vi "Litho Interpolater_shicheng.vi"(3 "Function generator":T1(array[cluster]) {"square wave duty cycle (%)" format="%0.2f"}, 4 "Lithography Data In":T2(array[cluster]), 5 "Distance":dbl) -> (0 "XY Graph":cluster{dbl[], "Y":dbl[]}(graph), 1 "Simulator Data Out":T3(array[cluster]), 2 "Lithography Data Out":T4(array[cluster]))   [LabVIEW 2013]
doc: "This VI takes lithography information as an input and interpolates points between and within patterns. It also maps voltages onto colors for the simulator."
uses:
  <vilib>/measure/NI_MABase.lvlib
panel:
  in  "generator index":dbl
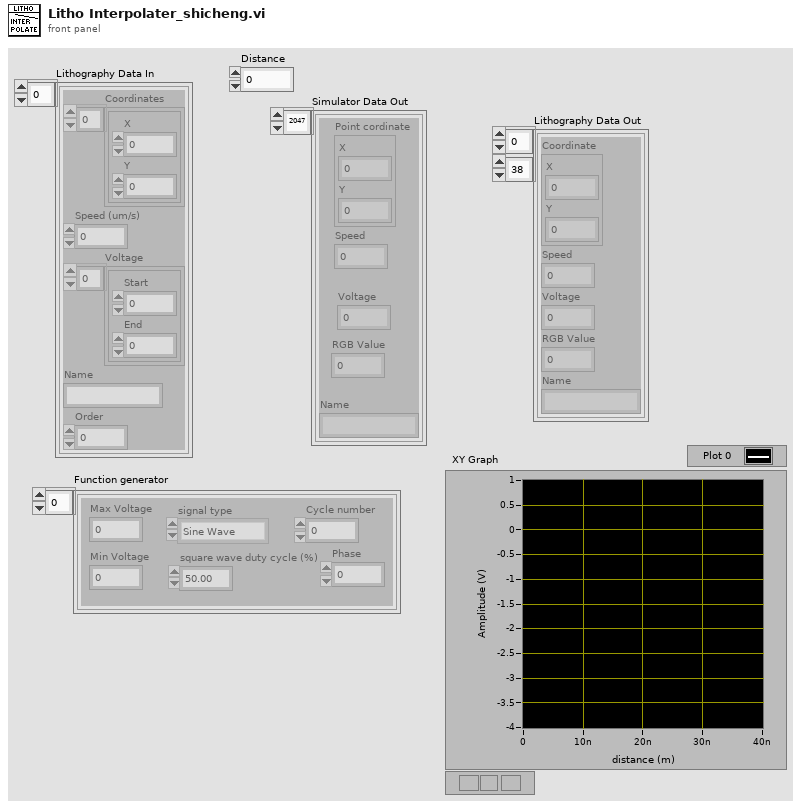
[diagram p1: front panel]
types:
  T1 = cluster{"Max Voltage":dbl, "Min Voltage":dbl, "signal type":enum16{"Sine Wave", "Triangle Wave", "Square Wave", "Sawtooth Wave"}, "square wave duty cycle (%)":dbl, "Cycle number":dbl, "Phase":dbl}[]
  T2 = cluster{"Coordinates":cluster{"X":dbl, "Y":dbl}[], "Speed (um/s)":dbl, "Voltage":cluster{"Start":dbl, "End":dbl}[], "Name":string, "Order":i32}[]
  T3 = cluster{"Point cordinate":cluster{"X":dbl, "Y":dbl}, "Speed":dbl, "Voltage":dbl, "RGB Value":i32, "Name":string}[]
  T4 = cluster{"Coordinate":cluster{"X":dbl, "Y":dbl}, "Speed":dbl, "Voltage":dbl, "RGB Value":i32, "Name":string}[][]
  T5 = cluster{"Point cordinate":cluster{"X":dbl, "Y":dbl}, "Speed":dbl, dbl, i32, "Name":string}[]
  T6 = cluster{"Coordinate":cluster{"X":dbl, "Y":dbl}, "Speed (um/s)":dbl, dbl, i32, "Name":string}[]
  T7 = cluster{"Point cordinate":cluster{"X":dbl, "Y":dbl}, "Speed":dbl, dbl, i32, "Name":string}
  T8 = cluster{"Coordinate":cluster{"X":dbl, "Y":dbl}, "Speed (um/s)":dbl, dbl, i32, "Name":string}
  T9 = cluster{"Max Voltage":dbl, "Min Voltage":dbl, "signal type":enum16{"Sine Wave", "Triangle Wave", "Square Wave", "Sawtooth Wave"}, "square wave duty cycle (%)":dbl, "Cycle number":dbl, "Phase":dbl}
  T10 = enum16{"Sine Wave", "Triangle Wave", "Square Wave", "Sawtooth Wave"}
  T11 = cluster{"Coordinate":cluster{"X":dbl, "Y":dbl}, "y":dbl, "y":dbl, i32, string}
  T12 = cluster{"Coordinate":cluster{"X":dbl, "Y":dbl}, "Speed (um/s)":dbl, "y":dbl, i32, "Name":string}[]
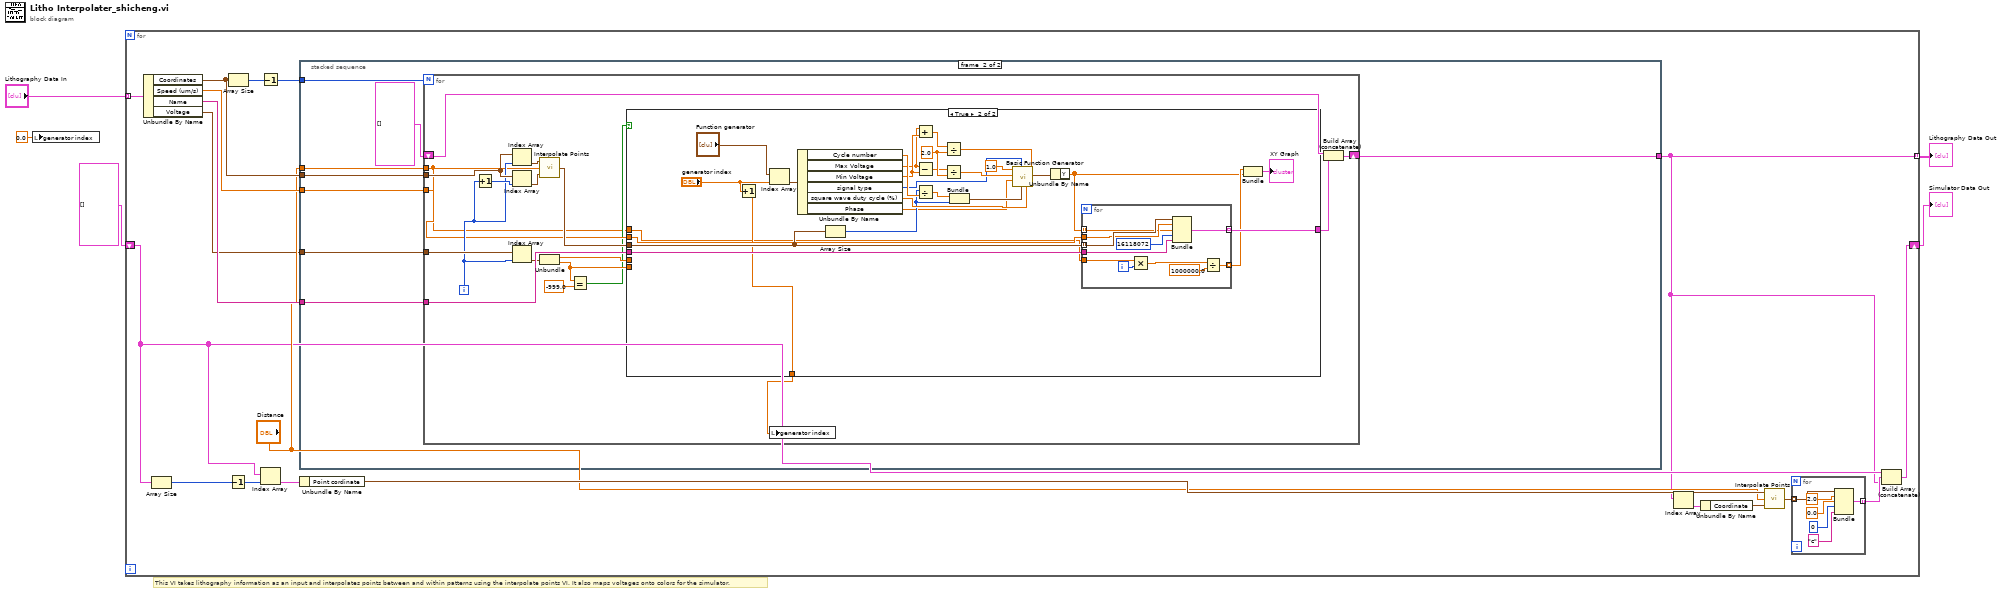
[diagram p0: block diagram]
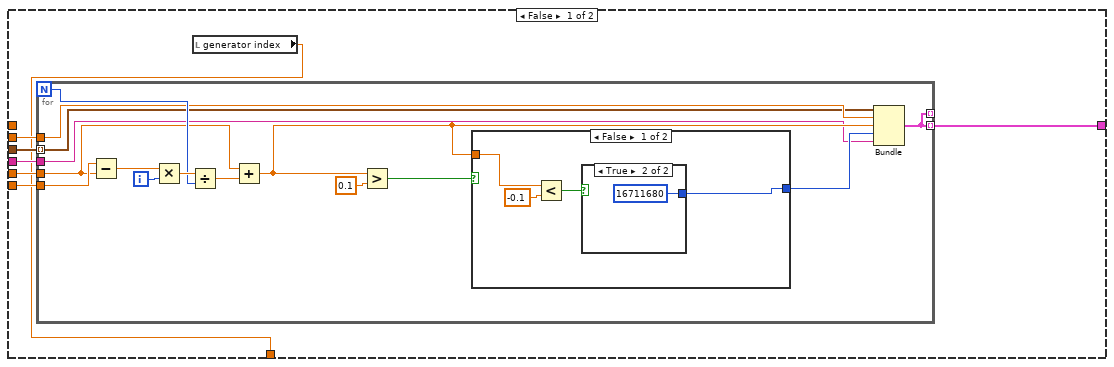
[diagram p3: hidden frame]
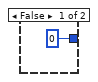
[diagram p4: hidden frame]
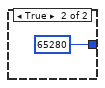
[diagram p5: hidden frame]
diagram:
  # "This VI takes lithography information as an input and interpolates points between and within patterns using the interpolate points VI. It also maps voltages onto colors for the simulator."
  n1 = local write "generator index"(0.0 ("generator index")) -> ()
  n2 = for {
    tunnel: "Lithography Data In" -> [w12] mode=indexing
    tunnel: [w9] -> w5 mode=indexing
    shift-right: [w19] -> w3
    shift-left: T5 [] -> [w14]
    n3 = Unbundle By Name(w12) -> ("Coordinates"=w22:cluster{"X":dbl, "Y":dbl}[], "Speed (um/s)"=w21:dbl, "Name"=w20:string, "Voltage"=w6:cluster{"Start":dbl, "End":dbl}[])
    n4 = Array Size(array=w14) -> (size(s)=w8:i32)
    n5 = Decrement(x=w8) -> (x-1=w7:i32)
    n6 = Array Size(array=w22) -> (size(s)=w24:i32)
    n7 = Index Array(array=w14, index=w7) -> (element=w13:T7)
    n8 = Decrement(x=w24) -> (x-1=w23:i32)
    n9 = stacked-sequence {
      tunnel: "Distance" -> [_ w38]
      tunnel: w23 -> [_ w37]
      tunnel: w22 -> [_ w36]
      tunnel: w21 -> [_ w34]
      tunnel: [_ w31] -> w9
      tunnel: w20 -> [_ w33]
      tunnel: w6 -> [_ w35]
      frame #0 {
      }
      frame #1 {
        n10 = for {
          N: w37 -> [_]
          tunnel: w38 -> [w39]
          tunnel: w36 -> [w56]
          tunnel: w35 -> [w53]
          tunnel: w34 -> [w50]
          tunnel: w33 -> [w49]
          shift-right: [w47] -> w31
          shift-left: T6 [] -> [w46]
          i -> [w52]
          n11 = Increment(x=w52) -> (x+1=w57:i32)
          n12 = Index Array(array=w56, index=w52) -> (element=w54:cluster{"X":dbl, "Y":dbl})
          n13 = Index Array(array=w56, index=w57) -> (element=w55:cluster{"X":dbl, "Y":dbl})
          n14 = Index Array(array=w53, index=w52) -> (element=w45:cluster{"Start":dbl, "End":dbl})
          n15 = call <vilib>:"Interpolate Points.vi"("End Point"=w55, "Distance between Points"=w39, "Start Point"=w54) -> ("Output Point Array"=w51:cluster{"X":dbl, "Y":dbl}[])
          n16 = Unbundle(w45) -> ("Start"=w44:dbl, "End"=w43:dbl)
          n17 = Equal?(x=w43, y=-999.0) -> (x = y?=w41:bool)
          n18 = case shown="True" w41 {
            tunnel: w51 -> [w64 w99]
            tunnel: w50 -> [w63 w114]
            tunnel: w49 -> [w62 w97]
            tunnel: [w61 w96] -> w48
            tunnel: w43 -> [w60 _]
            tunnel: w44 -> [w59 _]
            tunnel: [w58 w92] -> w40
            tunnel: w39 -> [_ w90]
            frame False {
              n19 = for {
                N -> [w75]
                tunnel: w64 -> [w66] mode=indexing
                tunnel: w63 -> [w74]
                tunnel: w59 -> [w72]
                tunnel: w60 -> [w79]
                tunnel: [w65] -> _ mode=indexing
                tunnel: w62 -> [w67]
                tunnel: [w65] -> w61 mode=indexing
                i -> [w77]
                n20 = Subtract(x=w79, y=w72) -> (x-y=w78:dbl)
                n21 = Multiply(x=w78, y=w77) -> (x*y=w76:dbl)
                n22 = Divide(x=w76, y=w75) -> (x/y=w73:dbl)
                n23 = Add(x=w72, y=w73) -> (x+y=w68:dbl)
                n24 = Greater?(x=w68, y=0.1) -> (0:w70:bool)
                n25 = case shown="False" w70 {
                  tunnel: [w83 65280] -> w69
                  tunnel: w68 -> [w81 _]
                  frame False {
                    n26 = Less?(x=w81, y=-0.1) -> (x < y?=w80:bool)
                    n27 = case shown="True" w80 {
                      tunnel: [0 16711680] -> w83
                      frame False {
                      }
                      frame True {
                      }
                    }
                  }
                  frame True {
                  }
                }
                n28 = Bundle("Coordinate"=w66, "Speed (um/s)"=w74, w68, w69, "Name"=w67) -> (w65:T8)  [unwired: 1 in]
              }
              n29 = local read "generator index"() -> (w58:dbl)
            }
            frame True {
              w108 = 2.0 ("y")
              n30 = Increment(x="generator index") -> (x+1=w92:dbl)
              n31 = Index Array(array="Function generator", index="generator index") -> (element=w101:T9)
              n32 = Unbundle By Name(w101) -> ("Cycle number"=w112:dbl, "Max Voltage"=w105:dbl, "Min Voltage"=w106:dbl, "signal type"=w104:T10, "square wave duty cycle (%)"=w110:dbl, "Phase"=w91:dbl)
              n33 = Array Size(array=w99) -> (size(s)=w98:i32)
              n34 = Add(x=w105, y=w106) -> (x+y=w102:dbl)
              n35 = Subtract(x=w105, y=w106) -> (x-y=w107:dbl)
              n36 = Divide(x=w98, y=w112) -> (x/y=w113:dbl)
              n37 = Divide(x=w102, y=w108) -> (x/y=w103:dbl)
              n38 = Divide(x=w107, y=w108) -> (x/y=w109:dbl)
              n39 = Bundle(w113, w98) -> (w111:cluster{dbl, i32})  [unwired: 1 in]
              n40 = call <vilib>:"Basic Function Generator.vi"("offset"=w103, "square wave duty cycle (%)"=w110, "sampling info"=w111, "signal type"=w104, "phase"=w91, "amplitude"=w109, "frequency"=1.0) -> ("signal out"=w94:waveform(dbl))  [unwired: 2 in, 2 out]
              n41 = Unbundle By Name(w94) -> ("Y"=w88:dbl[])
              n42 = for {
                tunnel: w99 -> [w125] mode=indexing
                tunnel: w114 -> [w124]
                tunnel: w88 -> [w123] mode=indexing
                tunnel: w97 -> [w121]
                tunnel: [w120] -> w96 mode=indexing
                tunnel: w90 -> [w118]
                tunnel: [w115] -> w89 mode=indexing
                i -> [w119]
                n43 = Multiply(x=w118, y=w119) -> (x*y=w117:dbl)
                n44 = Bundle("Coordinate"=w125, "Speed (um/s)"=w124, w123, 16118072, "Name"=w121) -> (w120:T8)  [unwired: 1 in]
                n45 = Divide(x=w117, y=1000000.0) -> (x/y=w115:dbl)
              }
              n46 = Bundle(w89, "Y"=w88) -> (→"XY Graph":cluster{dbl[], "Y":dbl[]})  [unwired: 1 in]
            }
          }
          n47 = local write "generator index"(w40) -> ()
          n48 = Build Array (concatenate)(w46, w48) -> (w47:T6)
        }
      }
    }
    n49 = Unbundle By Name(w13) -> ("Point cordinate"=w18:cluster{"X":dbl, "Y":dbl})
    n50 = Index Array(array=w9) -> (element=w15:T8)  [unwired: 1 in]
    n51 = Unbundle By Name(w15) -> ("Coordinate"=w17:cluster{"X":dbl, "Y":dbl})
    n52 = call <vilib>:"Interpolate Points.vi"("End Point"=w17, "Distance between Points"="Distance", "Start Point"=w18) -> ("Output Point Array"=w11:cluster{"X":dbl, "Y":dbl}[])
    n53 = for {
      tunnel: w11 -> [w30] mode=indexing
      tunnel: [w25] -> w10 mode=indexing
      n54 = Bundle("Coordinate"=w30, "y"=2.0, "y"=0.0, 0, "c") -> (w25:T11)  [unwired: 1 in]
    }
    n55 = Build Array (concatenate)(w14, w10, w9) -> (w19:T12)
  }
  "Lithography Data Out" <- w5
  "Simulator Data Out" <- w3
